vi "Remove Dataset Names.vi"(8 "error in (no error)":errorcluster, 10 "Dataset Names":string[](array[string])) -> (0 "error out":errorcluster, 2 "Name less Commands and Comments":string[](array[string]))   [LabVIEW 2016, in "LVtoITX.lvclass"]
uses:
  LVtoITX.lvclass
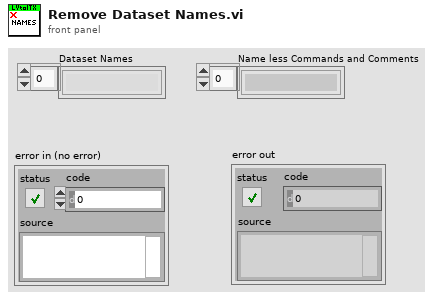
[diagram p1: front panel]
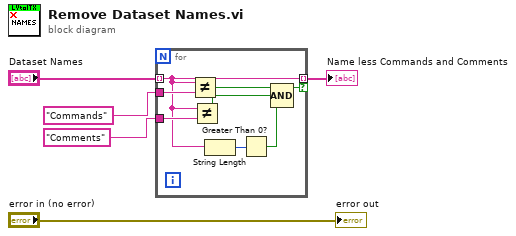
[diagram p0: block diagram]
diagram:
  n1 = for {
    tunnel: "Dataset Names" -> [w8] mode=indexing
    tunnel: [w8] -> w5 mode=indexing if=w9
    tunnel: "Commands" ("attrib name") -> [w11]
    tunnel: "Comments" ("attrib name") -> [w10]
    n2 = Not Equal?(x=w8, y=w11) -> (x != y?=w13:bool)
    n3 = Not Equal?(x=w8, y=w10) -> (x != y?=w12:bool)
    n4 = String Length(string=w8) -> (length=w7:i32)
    n5 = Greater Than 0?(x=w7) -> (x > 0?=w6:bool)
    n6 = Compound Arithmetic op=AND(w13, w12, w6) -> (w9:bool)
  }
  "Name less Commands and Comments" <- w5
  "error out" <- "error in (no error)"
